vi "REx - Send Command.vi"(0 "Remote Connection Handle in":T2, 7 "Command Data Element in":T1, 11 "error in (no error)":errorcluster) -> (4 "Remote Connection Handle out":T2, 8 "Command Data Element out":T1, 15 "error out":errorcluster)   [LabVIEW 2012, in "Alpha Cmd.lvclass"]
uses:
  Alpha Cmd.lvclass
  _REx/Components/Remote Connection Session/Typedefs/Session Handle.ctl
  _REx/Components/Remote Connection Session/Remote Connection Session.lvclass
  STYP - Command Data Element.ctl
  set Command Data Element.vi
  _REx/Components/REx Command Root/set Timeout.vi
  _REx/Components/REx Command Root/set Wait For Response.vi
  get Command Data Element.vi
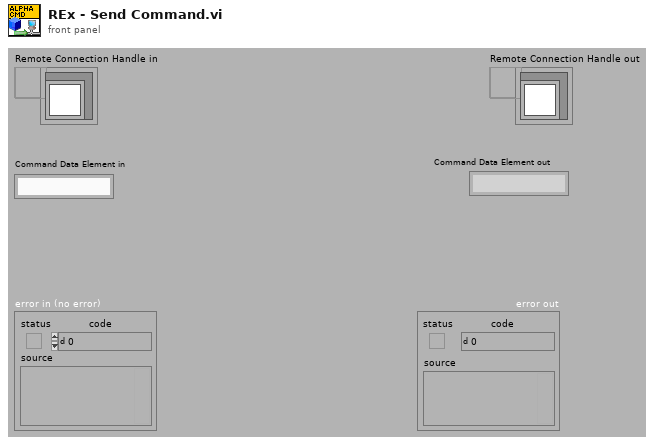
[diagram p1: front panel]
types:
  T1 = typedef "Alpha Cmd.lvclass/STYP - Command Data Element.ctl" = string
  T2 = typedef "REx.lvlib/Remote Connection Session.lvclass/Session Handle.ctl" = refnum<data-value>
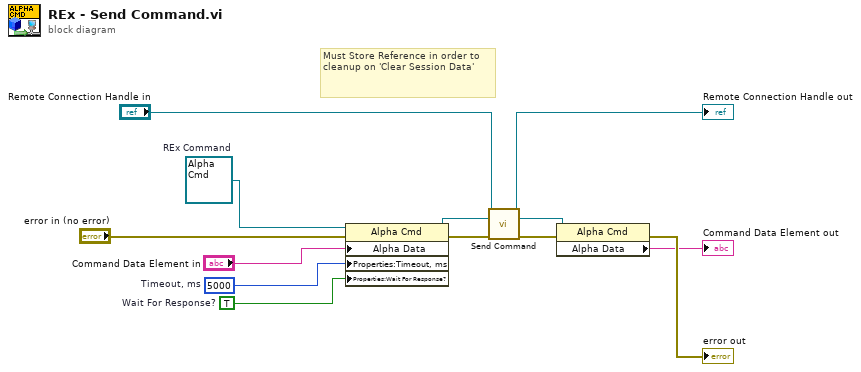
[diagram p0: block diagram]
diagram:
  w7 = TRUE  # Wait For Response?
  w11 = 5000  # Timeout, ms
  w10 = refnum<class "Alpha Cmd.lvclass"> refnum  # REx Command
  # "Must Store Reference in order to cleanup on 'Clear Session Data'"
  n1 = property class="Alpha Cmd"(reference=w10, error in="error in (no error)", "Alpha Data"="Command Data Element in", "Properties:Timeout, ms"=w11, "Properties:Wait For Response?"=w7) -> (reference out=w9:refnum<class "Alpha Cmd.lvclass">, error out=w8:errorcluster)
  n2 = call "Send Command.vi"("Session Handle in"="Remote Connection Handle in", "REx Command in"=w9, "error in (no error)"=w8) -> ("Session Handle out"=→"Remote Connection Handle out":T2, "REx Command out"=w6:refnum<class "Alpha Cmd.lvclass">, "error out"=w5:errorcluster)  [unwired: 10 in]
  n3 = property class="Alpha Cmd"(reference=w6, error in=w5) -> (error out=→"error out":errorcluster, "Alpha Data"=→"Command Data Element out":T1)  [unwired: 1 out]
